vi "Create G-CLI Sink.vi"(8 "error in (no error)":errorcluster, 11 "CLI Connection":refnum<class "CLI.lvclass">) -> (0 "error out":errorcluster)   [LabVIEW 2020, in "LV Logging.lvlib"]
uses:
  LV Logging.lvlib
  <vilib>/Wiresmith Technology/G CLI/CLI Class/CLI.lvclass
  G-CLI Sink/G-CLI Sink.lvclass
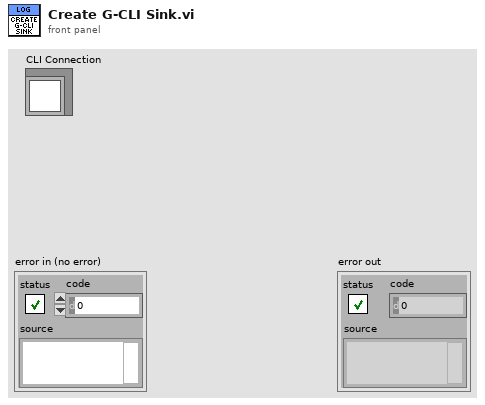
[diagram p1: front panel]
types:
  T1 = enum16{"Init", "Get Logger", "Register Sink", "Set Global Debug Level", "Get Sinks"}
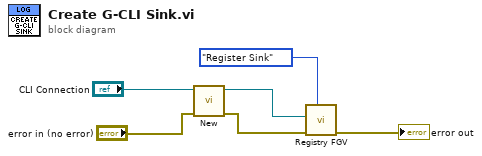
[diagram p0: block diagram]
diagram:
  n1 = call "New.vi"("error in (no error)"="error in (no error)", "CLI Connection"="CLI Connection") -> ("error out"=w3:errorcluster, "G-CLI Sink out"=w2:refnum<class "G-CLI Sink.lvclass">)  [unwired: 8 in]
  n2 = call "Registry FGV.vi"("State (Get Logger)"=T1."Register Sink", "error in (no error)"=w3, "Sink"=w2) -> ("error out"=→"error out":errorcluster)  [unwired: 5 in, 3 out]
